vi "step_MPB_sequence.vi"(8 "error in":errorcluster, 10 "default step":T3 {"data num" format="%.3f"}) -> (0 "error out":errorcluster, 2 "test results":T1)   [LabVIEW 2020]
uses:
  controls/MPB_step.ctl
  controls/MPB_step_type.ctl
  controls/test results.ctl
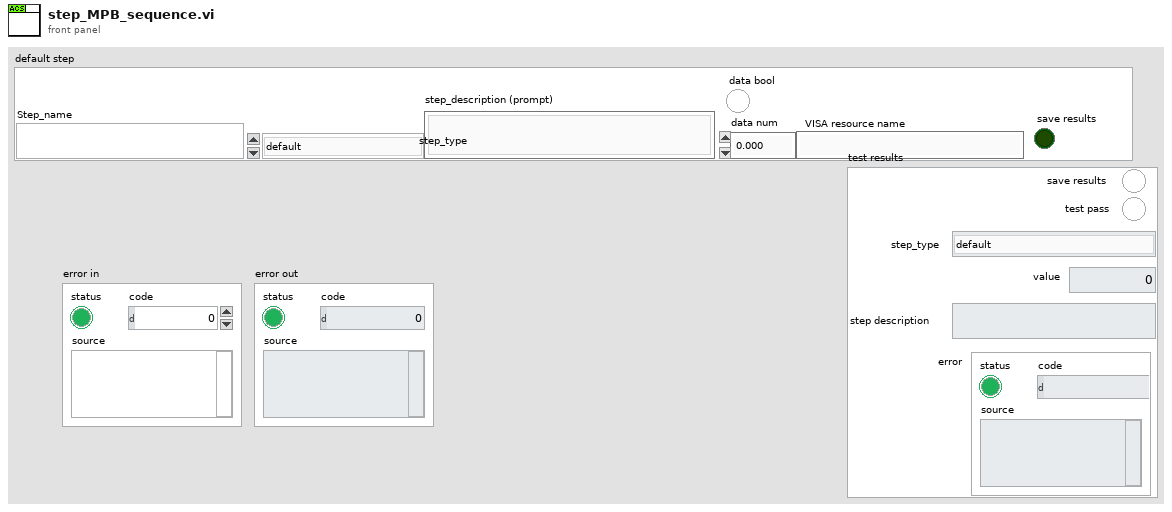
[diagram p1: front panel]
types:
  T1 = typedef "test results.ctl" = cluster{"test pass":bool, "step_type":T2, "value":dbl, "step description":string, "error":errorcluster, "save results":bool}
  T2 = typedef "MPB_step_type.ctl" = enum16{"default", "prompt", "sequence#", "12V_1_power supply on_off", "12V_2_power supply on_off", "set_hipot_V", "set_hipot_I_limit", "set_hipot_ramping (sec)", "set hipot_hold_time", "read_hipot_V", "read_hipot_I", "set_daq", "read_daq", "flash uds", "wait (sec)", "record_pass_fail", "ac_charge_test", "dc_400V_charging", "HAPS Heater Output", "HAPS Compressor Output", "stop_test", "error_exit"}
  T3 = typedef "MPB_step.ctl" = cluster{"VISA resource name":string, "data num":dbl, "step_description (prompt)":string, "save results":bool, "step_type":T2, "Step_name":string, "data bool":bool}
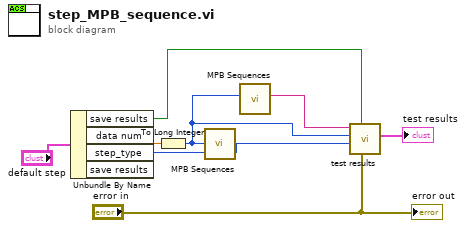
[diagram p0: block diagram]
diagram:
  n1 = Unbundle By Name("default step") -> ("save results"=w2:bool, "data num"=w4:dbl, "step_type"=w6:T2)  [unwired: 1 out]
  n2 = To Long Integer(number=w4) -> (32bit integer=w7:i32)
  n3 = call "MPB Sequences.vi"("sequence number"=w7) -> ()  [unwired: 10 in, 1 out]
  n4 = call "MPB Sequences.vi"("sequence number"=w7) -> ("(description) used in test"=w8:string)  [unwired: 10 in]
  n5 = call "test results.vi"("error"="error in", "save results"=w2, "step_type"=w6, "Numeric"=w7, "(description) used in test"=w8) -> ("test results"=→"test results":T1)  [unwired: 6 in]
  "error out" <- "error in"
